vi "crate_checking.vi"() -> ()   [LabVIEW 2025]
panel:
  in  "STOP":bool
  in  "Run this project":bool
  out "?":bool
  out "number":u32
  out "?":bool
  out "Crate's bottles":T1
  out "BOX":bool
  in  "amount of bottles":i32
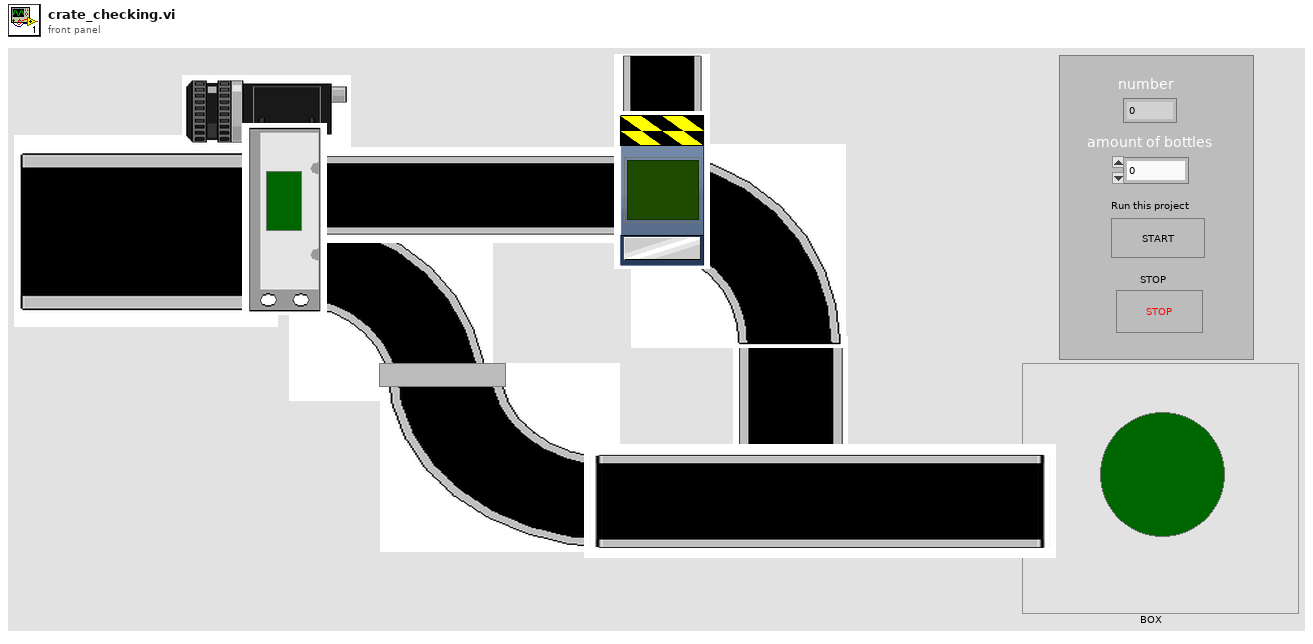
[diagram p1: front panel]
types:
  T1 = cluster{bool, bool, bool, bool, bool, bool, bool, bool, bool}
  T2 = cluster{"Boolean array[0]":bool, "Boolean array[1]":bool, "Boolean array[2]":bool, "Boolean array[3]":bool, "Boolean array[4]":bool, "Boolean array[5]":bool, "Boolean array[6]":bool, "Boolean array[7]":bool, "Boolean array[8]":bool}
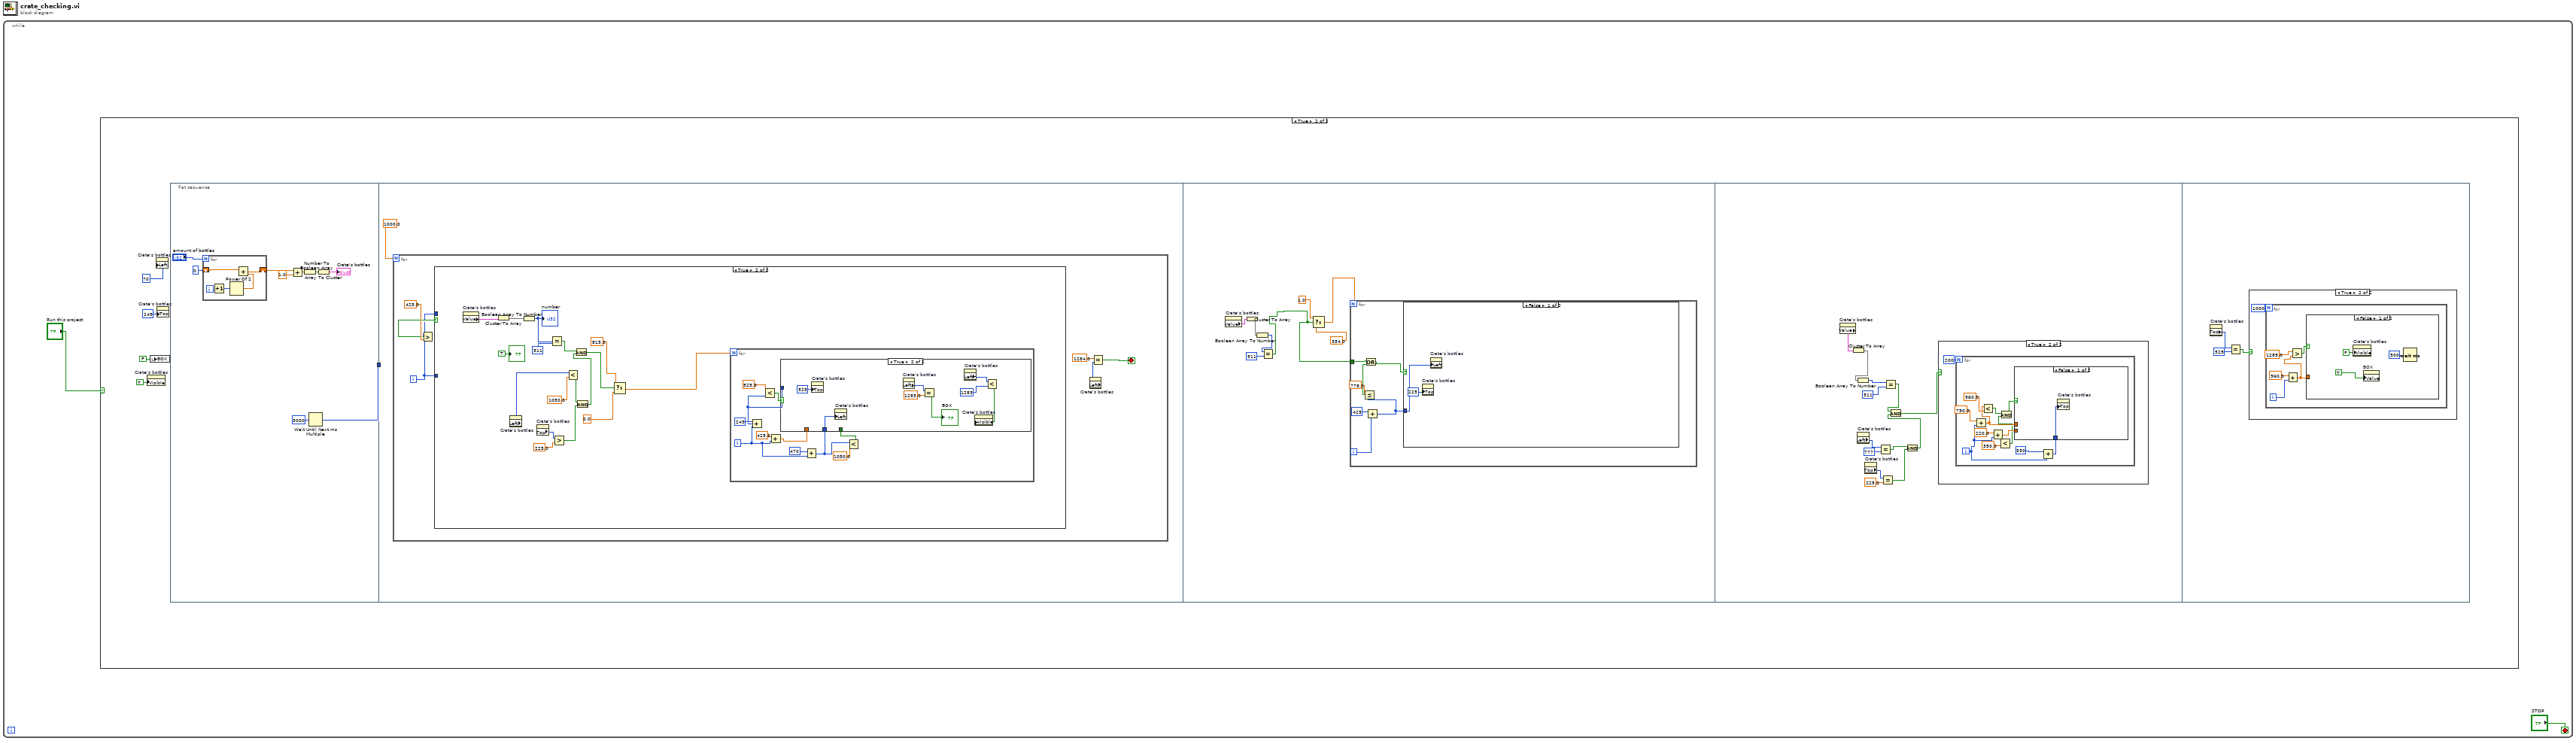
[diagram p0: block diagram]
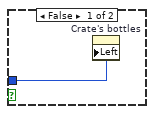
[diagram p3: hidden frame]
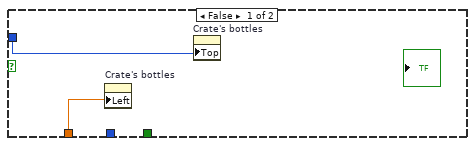
[diagram p4: hidden frame]
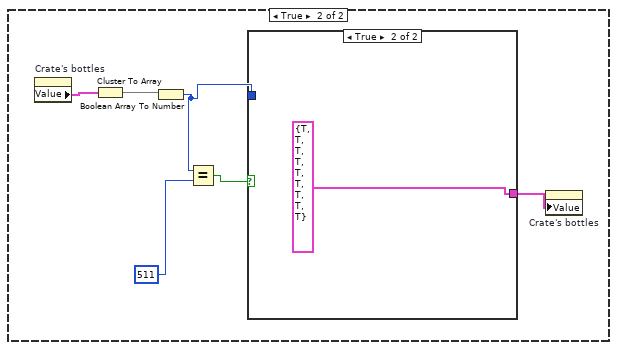
[diagram p5: hidden frame]
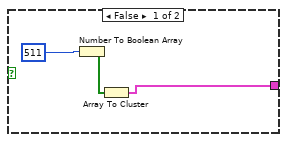
[diagram p6: hidden frame]
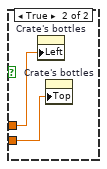
[diagram p8: hidden frame]
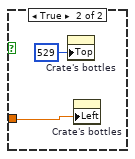
[diagram p10: hidden frame]
diagram:
  n1 = while {
    stop <- "STOP" stop-if-true
    n2 = case shown="True" "Run this project" {
      frame False {
      }
      frame True {
        n3 = property on="Crate's bottles" class="Clust (strict)"("Visible"=TRUE) -> ()  [unwired: 2 in, 2 out]
        n4 = local write "BOX"(FALSE ("BOX")) -> ()
        n5 = property on="Crate's bottles" class="Clust (strict)"("Left"=70 ("Position:Left")) -> ()  [unwired: 2 in, 2 out]
        n6 = property on="Crate's bottles" class="Clust (strict)"("Top"=249 ("Position:Top")) -> ()  [unwired: 2 in, 2 out]
        n7 = flat-sequence {
          tunnel: [w8] -> w7
          tunnel: w7 -> [_]
          frame #0 {
            n8 = for {
              N: "amount of bottles" -> [_]
              shift-right: [w20] -> w13
              shift-left: u32 0 -> [w21]
              i -> [w18]
              n9 = Increment(x=w18) -> (x+1=w17:i32)
              n10 = Power Of 2(x=w17) -> (2^x=w19:dbl)
              n11 = Add(x=w21, y=w19) -> (x+y=w20:dbl)
            }
            n12 = Add(x=w13, y=1.0) -> (x+y=w14:dbl)
            n13 = Number To Boolean Array(number=w14) -> (Boolean array=w15:bool[])
            n14 = Wait Until Next ms Multiple(millisecond multiple=u32 3000) -> (millisecond timer value=w8:u32)
            n15 = Array To Cluster(array=w15) -> (cluster=→"Crate's bottles":T2)
          }
          frame #1 {
            n16 = for {
              N: 1000.0 ("t") -> [_]
              i -> [w26]
              stop <- w23 stop-if-true
              n17 = Greater?(x=w26, y=425.0) -> (0:w27:bool)
              n18 = case shown="True" w27 {
                tunnel: w26 -> [w29 _]
                tunnel: w26 -> [_ _]
                frame False {
                  n19 = property on="Crate's bottles" class="Clust (strict)"("Left"=w29) -> ()  [unwired: 2 in, 2 out]
                }
                frame True {
                  n20 = property on="Crate's bottles" class="Clust (strict)"() -> ("Value"=w46:T1)  [unwired: 2 in, 2 out]
                  n21 = Cluster To Array(cluster=w46) -> (array=w45:bool[])
                  n22 = property on="Crate's bottles" class="Clust (strict)"() -> ("Left"=w37:i32)  [unwired: 2 in, 2 out]
                  n23 = Boolean Array To Number(Boolean array=w45) -> (number=w43:u32)
                  "number" <- w43
                  n24 = property on="Crate's bottles" class="Clust (strict)"() -> ("Top"=w33:i32)  [unwired: 2 in, 2 out]
                  n25 = Equal?(x=w43, y=u32 511) -> (x = y?=w35:bool)
                  n26 = Greater?(x=w33, y=225.0) -> (0:w32:bool)
                  n27 = Less?(x=w37, y=1050.0 ("x")) -> (x < y?=w31:bool)
                  n28 = And(x=w31, y=w32) -> (x .and. y?=w30:bool)
                  n29 = And(x=w35, y=w30) -> (x .and. y?=w38:bool)
                  n30 = Select(t=815.0, s=w38, f=0.0) -> (s? t:f=w39:dbl)
                  n31 = for {
                    N: w39 -> [_]
                    i -> [w50]
                    n32 = Add(x=249, y=w50) -> (x+y=w54:i32)
                    n33 = Less?(x=525.0, y=w54) -> (x < y?=w56:bool)
                    n34 = Add(x=425.0, y=w50) -> (x+y=w52:dbl)
                    n35 = Add(x=470, y=w50) -> (x+y=w48:i32)
                    n36 = Less?(x=w48, y=1050.0 ("x")) -> (x < y?=w51:bool)
                    n37 = case shown="True" w56 {
                      tunnel: w54 -> [w59 _]
                      tunnel: w52 -> [w58 _]
                      tunnel: w51 -> [_ _]
                      tunnel: w48 -> [_ w66]
                      frame False {
                        n38 = property on="Crate's bottles" class="Clust (strict)"("Left"=w58) -> ()  [unwired: 2 in, 2 out]
                        n39 = property on="Crate's bottles" class="Clust (strict)"("Top"=w59) -> ()  [unwired: 2 in, 2 out]
                      }
                      frame True {
                        n40 = property on="Crate's bottles" class="Clust (strict)"("Top"=525 ("Position:Top")) -> ()  [unwired: 2 in, 2 out]
                        n41 = property on="Crate's bottles" class="Clust (strict)"("Left"=w66) -> ()  [unwired: 2 in, 2 out]
                        n42 = property on="Crate's bottles" class="Clust (strict)"() -> ("Left"=w65:i32)  [unwired: 2 in, 2 out]
                        n43 = Equal?(x=w65, y=1283.0) -> (x = y?=→"BOX":bool)
                        n44 = property on="Crate's bottles" class="Clust (strict)"() -> ("Left"=w62:i32)  [unwired: 2 in, 2 out]
                        n45 = Less?(x=w62, y=1283) -> (x < y?=w60:bool)
                        n46 = property on="Crate's bottles" class="Clust (strict)"("Visible"=w60) -> ()  [unwired: 2 in, 2 out]
                      }
                    }
                  }
                  "?" <- TRUE
                }
              }
              n47 = property on="Crate's bottles" class="Clust (strict)"() -> ("Left"=w24:i32)  [unwired: 2 in, 2 out]
              n48 = Equal?(x=1284.0, y=w24) -> (x = y?=w23:bool)
            }
          }
          frame #2 {
            n49 = property on="Crate's bottles" class="Clust (strict)"() -> ("Value"=w73:T1)  [unwired: 2 in, 2 out]
            n50 = Cluster To Array(cluster=w73) -> (array=w74:bool[])
            n51 = Boolean Array To Number(Boolean array=w74) -> (number=w75:u32)
            n52 = Equal?(x=w75, y=u32 511) -> (x = y?=w68:bool)
            n53 = Select(t=1.0, s=w68, f=354.0) -> (s? t:f=w72:dbl)
            n54 = for {
              N: w72 -> [_]
              tunnel: w68 -> [w78]
              i -> [w81]
              n55 = Add(x=425, y=w81) -> (x+y=w79:i32)
              n56 = Less Or Equal?(x=778.0, y=w79) -> (x <= y?=w77:bool)
              n57 = Or(x=w78, y=w77) -> (x .or. y?=w76:bool)
              n58 = case shown="False" w76 {
                tunnel: w79 -> [w84 _]
                frame False {
                  n59 = property on="Crate's bottles" class="Clust (strict)"("Top"=225 ("Position:Top")) -> ()  [unwired: 2 in, 2 out]
                  n60 = property on="Crate's bottles" class="Clust (strict)"("Left"=w84) -> ()  [unwired: 2 in, 2 out]
                }
                frame True {
                  n61 = property on="Crate's bottles" class="Clust (strict)"() -> ("Value"=w89:T1)  [unwired: 2 in, 2 out]
                  n62 = Cluster To Array(cluster=w89) -> (array=w90:bool[])
                  n63 = Boolean Array To Number(Boolean array=w90) -> (number=w87:u32)
                  n64 = Equal?(x=w87, y=u32 511) -> (x = y?=w86:bool)
                  n65 = case shown="True" w86 {
                    tunnel: w87 -> [_ _]
                    tunnel: [w91 T2 {"Boolean array[0]"=TRUE, "Boolean array[1]"=TRUE, "Boolean array[2]"=TRUE, "Boolean array[3]"=TRUE, "Boolean array[4]"=TRUE, "Boolean array[5]"=TRUE, "Boolean array[6]"=TRUE, "Boolean array[7]"=TRUE, "Boolean array[8]"=TRUE} ("Boolean array")] -> w85
                    frame False {
                      n66 = Number To Boolean Array(number=511) -> (Boolean array=w92:bool[])
                      n67 = Array To Cluster(array=w92) -> (cluster=w91:T2)
                    }
                    frame True {
                    }
                  }
                  n68 = property on="Crate's bottles" class="Clust (strict)"("Value"=w85) -> ()  [unwired: 2 in, 2 out]
                }
              }
            }
          }
          frame #3 {
            n69 = property on="Crate's bottles" class="Clust (strict)"() -> ("Value"=w107:T1)  [unwired: 2 in, 2 out]
            n70 = Cluster To Array(cluster=w107) -> (array=w106:bool[])
            n71 = Boolean Array To Number(Boolean array=w106) -> (number=w105:u32)
            n72 = property on="Crate's bottles" class="Clust (strict)"() -> ("Left"=w102:i32)  [unwired: 2 in, 2 out]
            n73 = property on="Crate's bottles" class="Clust (strict)"() -> ("Top"=w98:i32)  [unwired: 2 in, 2 out]
            n74 = Equal?(x=w102, y=777) -> (x = y?=w100:bool)
            n75 = Equal?(x=w98, y=225.0) -> (x = y?=w97:bool)
            n76 = Equal?(x=w105, y=u32 511) -> (x = y?=w103:bool)
            n77 = And(x=w100, y=w97) -> (x .and. y?=w96:bool)
            n78 = And(x=w103, y=w96) -> (x .and. y?=w95:bool)
            n79 = case shown="True" w95 {
              frame False {
              }
              frame True {
                n80 = for {
                  N: 200 -> [_]
                  i -> [w111]
                  n81 = Add(x=790.0, y=w111) -> (x+y=w118:dbl)
                  n82 = Less?(x=w118, y=960.0 ("x")) -> (x < y?=w115:bool)
                  n83 = Add(x=220.0, y=w111) -> (x+y=w113:dbl)
                  n84 = Less?(x=w113, y=350.0) -> (x < y?=w112:bool)
                  n85 = And(x=w115, y=w112) -> (x .and. y?=w114:bool)
                  n86 = Add(x=330, y=w111) -> (x+y=w109:i32)
                  n87 = case shown="False" w114 {
                    tunnel: w118 -> [_ w123]
                    tunnel: w113 -> [_ w122]
                    tunnel: w109 -> [w121 _]
                    frame False {
                      n88 = property on="Crate's bottles" class="Clust (strict)"("Top"=w121) -> ()  [unwired: 2 in, 2 out]
                    }
                    frame True {
                      n89 = property on="Crate's bottles" class="Clust (strict)"("Left"=w123) -> ()  [unwired: 2 in, 2 out]
                      n90 = property on="Crate's bottles" class="Clust (strict)"("Top"=w122) -> ()  [unwired: 2 in, 2 out]
                    }
                  }
                }
              }
            }
          }
          frame #4 {
            n91 = property on="Crate's bottles" class="Clust (strict)"() -> ("Top"=w126:i32)  [unwired: 2 in, 2 out]
            n92 = Equal?(x=w126, y=529) -> (x = y?=w124:bool)
            n93 = case shown="True" w124 {
              frame False {
              }
              frame True {
                n94 = for {
                  N: 1000 -> [_]
                  i -> [w131]
                  n95 = Add(x=960.0, y=w131) -> (x+y=w128:dbl)
                  n96 = Greater?(x=1285.0, y=w128) -> (0:w129:bool)
                  n97 = case shown="False" w129 {
                    tunnel: w128 -> [_ w137]
                    frame False {
                      n98 = property on="Crate's bottles" class="Clust (strict)"("Visible"=FALSE) -> ()  [unwired: 2 in, 2 out]
                      n99 = property on="BOX" class="Bool (strict)"("Value"=TRUE ("BOX")) -> ()  [unwired: 2 in, 2 out]
                      n100 = Wait (ms)(milliseconds to wait=u32 500) -> ()  [unwired: 1 out]
                    }
                    frame True {
                      n101 = property on="Crate's bottles" class="Clust (strict)"("Top"=529 ("Position:Top")) -> ()  [unwired: 2 in, 2 out]
                      n102 = property on="Crate's bottles" class="Clust (strict)"("Left"=w137) -> ()  [unwired: 2 in, 2 out]
                    }
                  }
                }
              }
            }
          }
        }
      }
    }
  }
